vi "CrawlingState.vi"(8 "error in (no error)":errorcluster, 9 "Cluster in":T2, 10 "Enum in":T1, 11 "Actual Start [i]":i64) -> (0 "error out":errorcluster, 2 "Cluster out":T2, 3 "Enum":T1)   [LabVIEW 2018]
uses:
  Type_Def/Type_Def Actuator Controls.ctl
  Type_Def/Type_Def ControlState.ctl
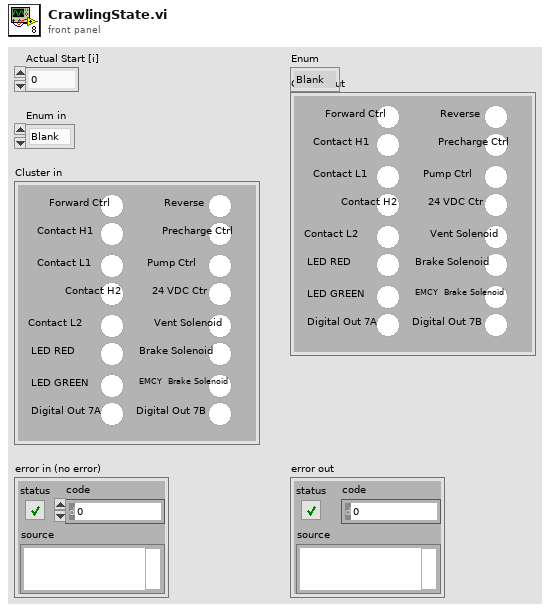
[diagram p1: front panel]
types:
  T1 = typedef "Type_Def ControlState.ctl" = enum16{"Blank", "Systems Check", "Idle", "Ready", "Pushing", "CrawlingPrecharge", "Braking", "Fault", "Boot Up", "Unpowered", "Crawling", "Shutdown", "Service Push", "Service Wait", "Vent", "Precharge", "Cooldown"}
  T2 = typedef "Type_Def Actuator Controls.ctl" = cluster{"Reverse ":bool, "Precharge Ctrl":bool, "Pump Ctrl":bool, "24 VDC Ctr":bool, "Vent Solenoid":bool, "Brake Solenoid":bool, "EMCY  Brake Solenoid":bool, "Digital Out 7B ":bool, "Forward Ctrl":bool, "Contact H1":bool, "Contact L1":bool, "Contact H2":bool, "Contact L2 ":bool, "LED RED":bool, "LED GREEN":bool, " Digital Out 7A":bool}
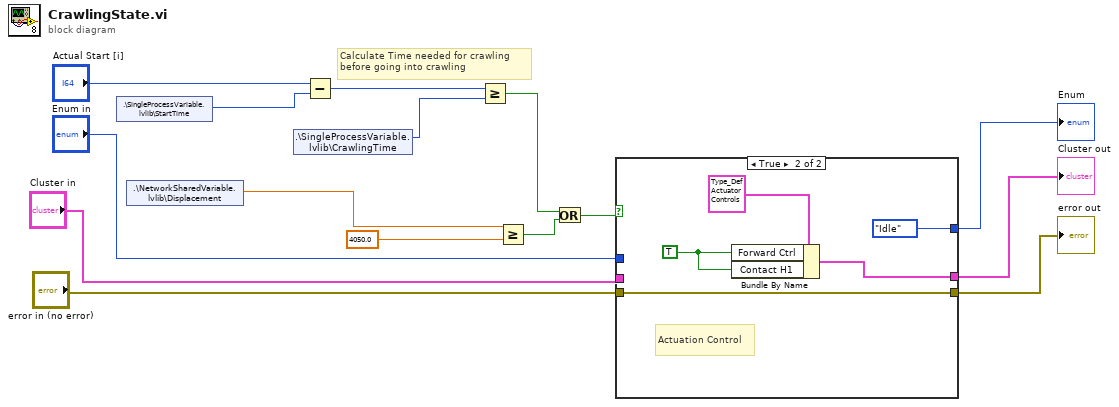
[diagram p0: block diagram]
diagram:
  # "Calculate Time needed for crawling \nbefore going into crawling"
  n1 = shared-variable ".\\SingleProcessVariable.lvlib\\StartTime"() -> (w8:i64)  [unwired: 1 in, 1 out]
  n2 = shared-variable ".\\NetworkSharedVariable.lvlib\\Displacement"() -> (w14:dbl)  [unwired: 1 in, 1 out]
  n3 = shared-variable ".\\SingleProcessVariable.lvlib\\CrawlingTime"() -> (w15:i64)  [unwired: 1 in, 1 out]
  n4 = Subtract(x="Actual Start [i]", y=w8) -> (x-y=w9:i64)
  n5 = Greater Or Equal?(x=w9, y=w15) -> (x >= y?=w10:bool)
  n6 = Greater Or Equal?(x=w14, y=4050.0) -> (x >= y?=w12:bool)
  n7 = Or(x=w10, y=w12) -> (x .or. y?=w13:bool)
  n8 = case shown="True" w13 {
    tunnel: "Enum in" -> [w18 _]
    tunnel: [w18 Type_Def_ControlState."Idle"] -> w2
    tunnel: "Cluster in" -> [w17 _]
    tunnel: [w17 w22] -> w4
    tunnel: [w16 w21] -> w5
    tunnel: "error in (no error)" -> [w16 w21]
    frame False {
    }
    frame True {
      w20 = TRUE ("Brake Valve")
      # "Actuation Control"
      n9 = Bundle By Name(cluster=T2 {"Reverse "=FALSE, "Precharge Ctrl"=FALSE, "Pump Ctrl"=FALSE, "24 VDC Ctr"=FALSE, "Vent Solenoid"=FALSE, "Brake Solenoid"=FALSE, "EMCY  Brake Solenoid"=FALSE, "Digital Out 7B "=FALSE, "Forward Ctrl"=FALSE, "Contact H1"=FALSE, "Contact L1"=FALSE, "Contact H2"=FALSE, "Contact L2 "=FALSE, "LED RED"=FALSE, "LED GREEN"=FALSE, " Digital Out 7A"=FALSE} ("Cluster in 2"), "Forward Ctrl"=w20, "Contact H1"=w20) -> (w22:T2)
    }
  }
  "error out" <- w5
  "Cluster out" <- w4
  "Enum" <- w2
